vi "RawHeader.vi"(0 "Tester":string="C Bradshaw", 1 "test request":string, 2 "purpose of test":string, 3 "varnames":string[](array[string]), 5 "build file":string, 9 "Comments on Test":string, 11 "Spreadsheet Data":string, 12 "units":string[](array[string]), 14 "Root Path":path) -> (4 "File Path":path, 15 "raw data filename string":string)   [LabVIEW 2017]
panel:
  # "Header"
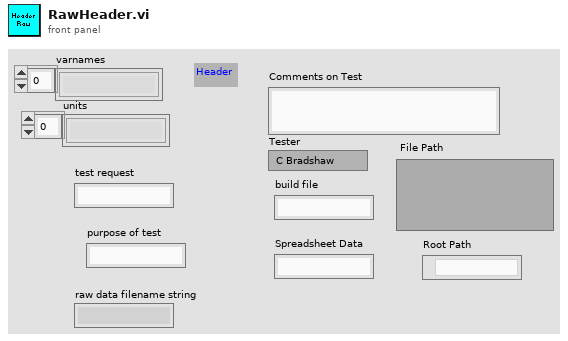
[diagram p1: front panel]
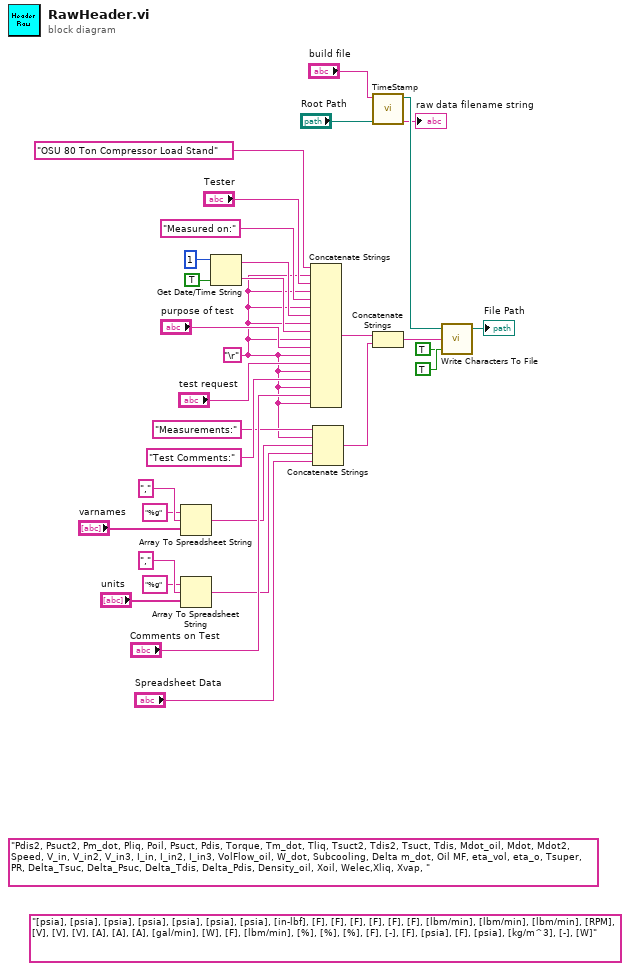
[diagram p0: block diagram]
diagram:
  (unwired) "[psia], [psia], [psia], [psia], [psia], [psia], [psia], [in-lbf], [F], [F], [F], [F], [F], [F], [lbm/min], [lbm/min], [lbm/min], [RPM], [V], [V], [V], [A], [A], [A], [gal/min], [W], [F], [lbm/min], [%], [%], [%], [F], [-], [F], [psia], [F], [psia], [kg/m^3], [-], [W]"
  (unwired) "Pdis2, Psuct2, Pm_dot, Pliq, Poil, Psuct, Pdis, Torque, Tm_dot, Tliq, Tsuct2, Tdis2, Tsuct, Tdis, Mdot_oil, Mdot, Mdot2, Speed, V_in, V_in2, V_in3, I_in, I_in2, I_in3, VolFlow_oil, W_dot, Subcooling, Delta m_dot, Oil MF, eta_vol, eta_o, Tsuper, PR, Delta_Tsuc, Delta_Psuc, Delta_Tdis, Delta_Pdis, Density_oil, Xoil, Welec,Xliq, Xvap, "
  w2 = "\r"
  n1 = Array To Spreadsheet String(delimiter (Tab)=",", array="varnames", 3:"%g" ("format string")) -> (spreadsheet string=w13:string)
  n2 = Array To Spreadsheet String(delimiter (Tab)=",", array="units", 3:"%g" ("format string")) -> (spreadsheet string=w6:string)
  n3 = Get Date/Time String(date format (0)=1, want seconds? (F)=TRUE) -> (date string=w26:string, time string=w25:string)  [unwired: 1 in]
  n4 = Concatenate Strings("OSU 80 Ton Compressor Load Stand", w2, "Tester", w2, "Measured on:", w2, w26, w2, w25, w2, "purpose of test", w2, "test request", w2, "Test Comments:", w2, "Comments on Test", w2) -> (w21:string)
  n5 = Concatenate Strings("Measurements:", w2, w13, w6, "Spreadsheet Data") -> (w20:string)
  n6 = call "TimeStamp.vi"("Root Path"="Root Path", "Build Name"="build file") -> ("filename string"=→"raw data filename string":string, "File Path"=w15:path)  [unwired: 7 in, 1 out]
  n7 = Concatenate Strings(w21, w20) -> (w19:string)
  n8 = call <vilib>:"Write Characters To File.vi"("convert eol? (no:F)"=TRUE, "append to file? (new file:F)"=TRUE, "character string"=w19, "file path (dialog if empty)"=w15) -> ("new file path (Not A Path if cancelled)"=→"File Path":path)  [unwired: 1 in]
